vi "Gaussian surface data.vi"(4 "Yend":dbl=1.1, 5 "output cluster":T1, 6 "Ystart":dbl=0.2, 7 "VI Refnum":refnum<vi>, 8 "noise sigma":dbl=0.05, 9 "Xend":dbl=0.5, 10 "Xstart":dbl, 11 "a":dbl[](array[numeric])) -> (0 "error out":errorcluster, 2 "X":dbl[](array[numeric]), 3 "Noisy 2D Gaussian surface data":dbl[](array[numeric]))   [LabVIEW 2023]
doc: "Generate noisy Gaussian surface data."
uses:
  <vilib>/Native 3D Graph/xcontrol/3DPC_SurfacePlot.xctl
  <vilib>/Analysis/1siggen.llb/Ramp Pattern by Samples.vi
  <vilib>/Analysis/NI_AALBase.lvlib
  <vilib>/Native 3D Graph/classes/Base Datatype.lvclass
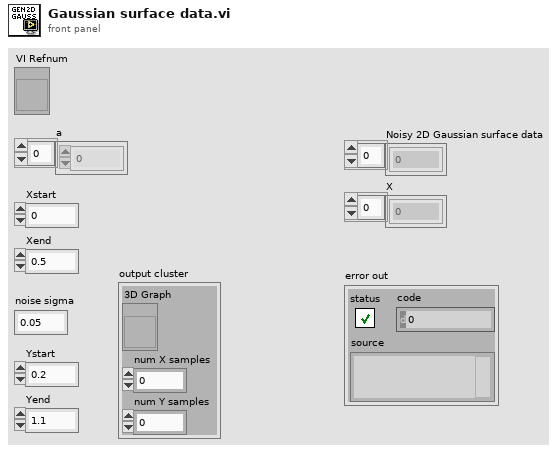
[diagram p1: front panel]
types:
  T1 = cluster{"3D Graph":refnum<vi>, "num X samples":i32, "num Y samples":i32}
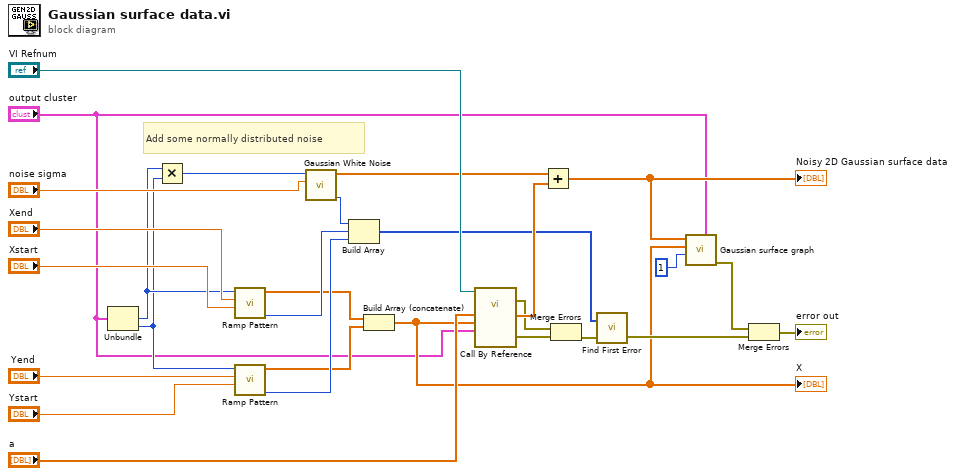
[diagram p0: block diagram]
diagram:
  # "Add some normally distributed noise"
  n1 = Unbundle("output cluster") -> ("num X samples"=w10:i32, "num Y samples"=w9:i32)  [unwired: 1 out]
  n2 = Multiply(x=w10, y=w9) -> (x*y=w21:i32)
  n3 = call-poly <vilib>:"Ramp Pattern.vi"("start"="Xstart", "end"="Xend", "samples"=w10) -> ("error"=w27:i32, "Ramp Pattern"=w16:dbl[])  [unwired: 7 in]
  n4 = call-poly <vilib>:"Ramp Pattern.vi"("start"="Ystart", "end"="Yend", "samples"=w9) -> ("error"=w26:i32, "Ramp Pattern"=w15:dbl[])  [unwired: 7 in]
  n5 = call <vilib>:"Gaussian White Noise.vi"("standard deviation"="noise sigma", "samples"=w21) -> ("error"=w28:i32, "Gaussian noise pattern"=w22:dbl[])  [unwired: 8 in]
  n6 = Build Array(w28, w27, w26) -> (w12:i32[])
  n7 = Build Array (concatenate)(w16, w15) -> (w7:dbl[])
  "X" <- w7
  n8 = call-by-ref "?"(reference="VI Refnum", "data"="output cluster", "X"=w7, "a"="a") -> (error out=w1:errorcluster, 0:"error out"=w13:errorcluster, "f(X,a)"=w14:dbl[])  [unwired: 2 in, 2 out]
  n9 = Add(x=w22, y=w14) -> (x+y=w8:dbl[])
  "Noisy 2D Gaussian surface data" <- w8
  n10 = Merge Errors(w1, w13) -> (w2:errorcluster)
  n11 = call <vilib>:"Find First Error.vi"("error in (no error)"=w2, "error codes"=w12) -> ("error out"=w11:errorcluster)  [unwired: 1 in, 2 out]
  n12 = call "Gaussian surface graph.vi"("output cluster"="output cluster", "plot number (1)"=1, "X"=w7, "Y"=w8) -> ("error out"=w4:errorcluster)  [unwired: 7 out]
  n13 = Merge Errors(w4, w11) -> (→"error out":errorcluster)
